vi "Highlight Selected Row in Table Control 2012 NIVerified.vi"() -> ()   [LabVIEW 2015]
doc: "This example lets you highlight a row based on which row a user clicks on. It changes the background color and then changes it back to blank when another row is clicked on."
uses:
  <vilib>/addons/database/Connection.llb/DB Tools Open Connec (Path).vi
  D:/TFS-Labview/Low Level Projects/TCSS Project/Global Variable/BalancingSubsystem_TCSS.vi
  D:/TFS-Labview/Low Level Projects/TCSS Project/TCSS/Sub VI/SQL_DB_Control/Logic/Class/SQL_DB_Control_class/SQL_DB_Control.lvclass
  <vilib>/addons/database/NI_Database_API.lvlib
panel:
  in  "?":bool
  out "Database Information":string[][](table)
  in  "stop":bool
  # "Overview: This example demonstrates a common practice of dealing with Tables programmatically,which lets you highlight a row based on which row a user clicks on. \nRequirements: LabVIEW 2012 (or compatible)\nInstruction:\n1. Run the VI\n2. Click on a row to highlight it."
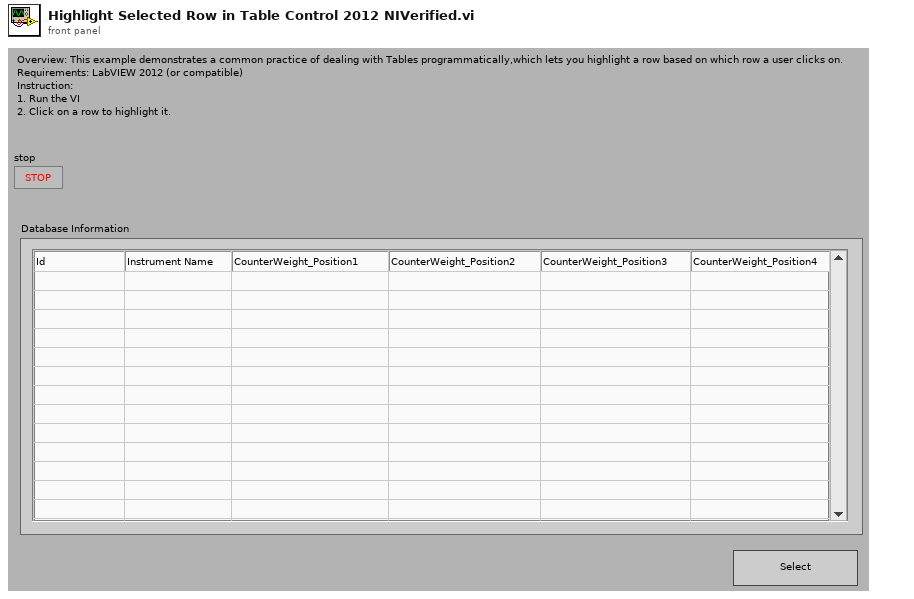
[diagram p1: front panel]
types:
  T1 = typedef "NI_Database_API.lvlib/Conn ObjectReference.ctl" = refnum<k1>
  T2 = typedef "LVRowAndColumnTypeDef.ctl" = cluster{"Row":i32, "Column":i32}
  T3 = cluster{"ControlScheme":cluster{"ID":i32, "Cold Start":bool, "Configuration":bool, "Start":bool, "Pointing/Tracking":bool, "Standby":bool, "Stop":bool, "Shutdown":bool, "Start Calibration":bool, "Start Maintenance":bool, "Status":i16, "Time ":timestamp}, "ControllerConfig":cluster{"ID":i32, "K_P Config":u64, "K_I Config":u64, "K_D Config":u64, "PID_Limit":u64, "Feedforward":u64, "Feedforward Tune":u64, "Output_Limit":u64, "Status":i16, "Time ":timestamp}, "BalancingMotor-All":cluster{"BalancingMotor-00":cluster{"ID":i32, "Target Position":u64, "Target Velocity":u64, "Enable":bool, "Direction":bool, "Brake":bool, "Built-In Encoder":u64, "Brake Voltage FB":bool, "Brake Current FB":u64, "Up Limit Switch":bool, "Down Limit Switch":bool, "LinearScale":u64, "Status":i16, "Time ":timestamp}, "BalancingMotor-01":cluster{"ID":i32, "Target Position":u64, "Target Velocity":u64, "Enable":bool, "Direction":bool, "Brake":bool, "Built-In Encoder":u64, "Brake Voltage FB":bool, "Brake Current FB":u64, "Up Limit Switch":bool, "Down Limit Switch":bool, "LinearScale":u64, "Status":i16, "Time ":timestamp}, "BalancingMotor-02":cluster{"ID":i32, "Target Position":u64, "Target Velocity":u64, "Enable":bool, "Direction":bool, "Brake":bool, "Built-In Encoder":u64, "Brake Voltage FB":bool, "Brake Current FB":u64, "Up Limit Switch":bool, "Down Limit Switch":bool, "LinearScale":u64, "Status":i16, "Time ":timestamp}, "BalancingMotor-03":cluster{"ID":i32, "Target Position":u64, "Target Velocity":u64, "Enable":bool, "Direction":bool, "Brake":bool, "Built-In Encoder":u64, "Brake Voltage FB":bool, "Brake Current FB":u64, "Up Limit Switch":bool, "Down Limit Switch":bool, "LinearScale":u64, "Status":i16, "Time ":timestamp}}, "BalancingControlCommand":cluster{"Start":bool, "Park":bool, " Stop":bool, "Configuration":bool}}
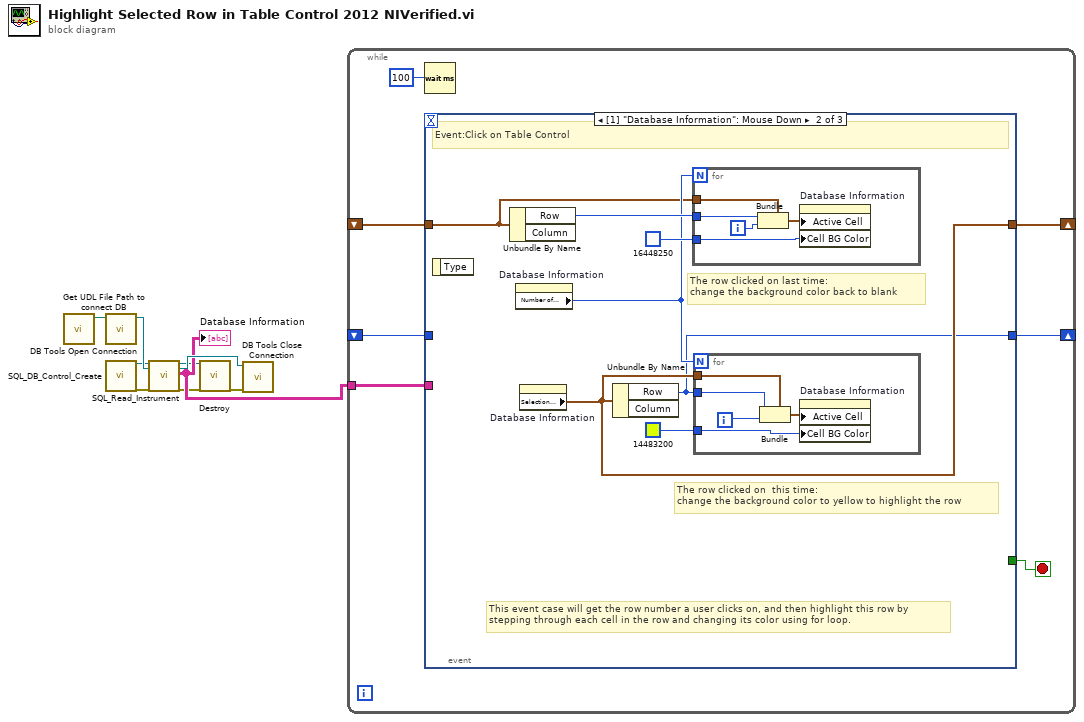
[diagram p0: block diagram]
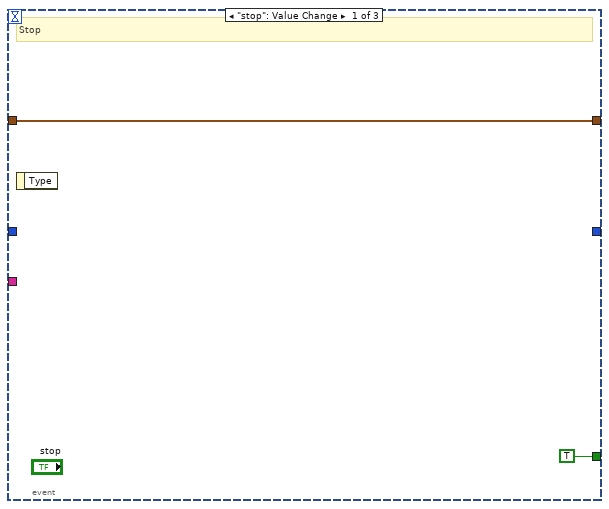
[diagram p2: hidden frame]
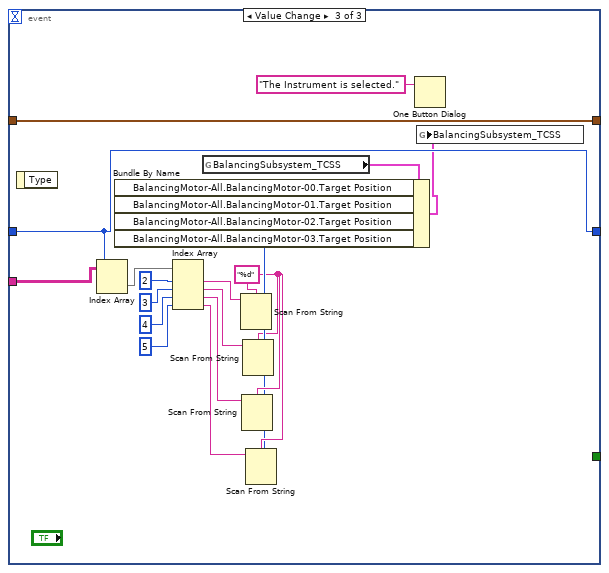
[diagram p3: hidden frame]
diagram:
  n1 = call "Get UDL File Path to connect DB.vi"() -> ("UDL file path"=w7:path)  [unwired: 11 in]
  n2 = call-poly <vilib>:"DB Tools Open Connection.vi"("connection information"=w7) -> ("connection reference"=w8:T1)  [unwired: 7 in, 1 out]
  n3 = call "SQL_DB_Control_Create.vi"() -> ("reference out"=w6:refnum<class "SQL_DB_Control.lvclass">, "error out"=w5:errorcluster)  [unwired: 18 in]
  n4 = call-dynamic "SQL_Read_Instrument.vi"("reference in"=w6, "connection reference in"=w8, "error in (no error)"=w5) -> ("reference out"=w2:refnum<class "SQL_DB_Control.lvclass">, "connection reference out"=w9:T1, "Instrument"=w4:string[][], "error out"=w3:errorcluster)  [unwired: 13 in]
  "Database Information" <- w4
  n5 = call-dynamic "Destroy.vi"("reference in"=w2, "error in (no error)"=w3) -> ("error out"=w1:errorcluster)  [unwired: 16 in, 1 out]
  n6 = call <vilib>:"DB Tools Close Connection.vi"("error in (no error)"=w1, "connection reference"=w9) -> ()  [unwired: 5 in, 1 out]
  n7 = while {
    shift-right: [w15] -> _
    shift-left: _ -> [w14]
    tunnel: w4 -> [w12]
    shift-right: [w11] -> _
    shift-left: _ -> [w10]
    stop <- w13 stop-if-true
    n8 = Wait (ms)(milliseconds to wait=u32 100) -> ()  [unwired: 1 out]
    n9 = event shown="[1] \"Database Information\": Mouse Down" {
      selector: _ -> [_ _ _]
      dyn-events: _ -> [_ _ _]
      timeout: _ -> [_ _ _]
      tunnel: [w18 w20 w38] -> w15
      tunnel: w14 -> [w18 w21 w38]
      tunnel: [TRUE _ _] -> w13
      tunnel: w12 -> [_ _ w40]
      tunnel: [_ w19 w39] -> w11
      tunnel: w10 -> [_ _ w39]
      event "stop": Value Change {
        # "Stop"
        n10 = event-data() -> ()  [unwired: 1 in, 1 out]
      }
      event "Database Information": Mouse Down {
        # "This event case will get the row number a user clicks on, and then highlight this row by \nstepping through each cell in the row and changing its color using for loop."
        # "The row clicked on  this time:\nchange the background color to yellow to highlight the row"
        # "The row clicked on last time:\nchange the background color back to blank"
        # "Event:Click on Table Control"
        n11 = event-data() -> ()  [unwired: 1 in, 1 out]
        n12 = Unbundle By Name(w21) -> ("Row"=w24:i32)  [unwired: 1 out]
        n13 = property on="Database Information" class="Tbl (strict)"() -> ("Number of Columns"=w22:u32)  [unwired: 2 in, 2 out]
        n14 = property on="Database Information" class="Tbl (strict)"() -> ("Selection Start"=w20:T2)  [unwired: 2 in, 2 out]
        n15 = Unbundle By Name(w20) -> ("Row"=w19:i32)  [unwired: 1 out]
        n16 = for {
          N: w22 -> [_]
          tunnel: u32 16448250 -> [w30]
          tunnel: w21 -> [w29]
          tunnel: w24 -> [w28]
          i -> [w27]
          n17 = Bundle(cluster=w29, "Row"=w28, "Column"=w27) -> (w26:T2)
          n18 = property on="Database Information" class="Tbl (strict)"("Active Cell"=w26, "Cell BG Color"=w30) -> ()  [unwired: 2 in, 2 out]
        }
        n19 = for {
          N: w22 -> [_]
          tunnel: u32 14483200 -> [w35]
          tunnel: w20 -> [w34]
          tunnel: w19 -> [w33]
          i -> [w32]
          n20 = Bundle(cluster=w34, "Row"=w33, "Column"=w32) -> (w31:T2)
          n21 = property on="Database Information" class="Tbl (strict)"("Active Cell"=w31, "Cell BG Color"=w35) -> ()  [unwired: 2 in, 2 out]
        }
      }
      event Value Change {
        w45 = "%d" ("format string")
        n22 = event-data() -> ()  [unwired: 1 in, 1 out]
        n23 = Index Array(array=w40, index (row)=w39) -> (element=w50:string[])  [unwired: 1 in]
        n24 = Index Array(array=w50, index #1=2, index #2=3 ("index"), index #3=4 ("index"), index #4=5 ("index")) -> (element #1=w49:string, element #2=w47:string, element #3=w42:string, element #4=w41:string)
        n25 = global read "BalancingSubsystem_TCSS.vi" "BalancingSubsystem_TCSS"() -> (w55:T3)
        n26 = Scan From String(format string=w45, input string=w49) -> (output 1=w48:i32)  [unwired: 3 in, 3 out]
        n27 = Scan From String(format string=w45, input string=w42) -> (output 1=w44:i32)  [unwired: 3 in, 3 out]
        n28 = Scan From String(format string=w45, input string=w47) -> (output 1=w46:i32)  [unwired: 3 in, 3 out]
        n29 = Scan From String(format string=w45, input string=w41) -> (output 1=w43:i32)  [unwired: 3 in, 3 out]
        n30 = Bundle By Name(cluster=w55, "BalancingMotor-All.BalancingMotor-00.Target Position"=w48, "BalancingMotor-All.BalancingMotor-01.Target Position"=w46, "BalancingMotor-All.BalancingMotor-02.Target Position"=w44, "BalancingMotor-All.BalancingMotor-03.Target Position"=w43) -> (w37:T3)
        n31 = One Button Dialog(message="The Instrument is selected.") -> ()  [unwired: 1 in, 1 out]
        n32 = global write "BalancingSubsystem_TCSS.vi" "BalancingSubsystem_TCSS"(w37) -> ()
      }
    }
  }
